vi "Super Market Billing System.vi"() -> ()   [LabVIEW 2021]
panel:
  in  "Tab Control":enum32{"Page 1", "Page 2"}(tab)
  in  "Refresh Button":bool
  in  "Password":string
  in  "User Name":string
  out "Result":dbl
  in  "Number 2":dbl
  in  "Number 1":dbl
  in  "stop":bool
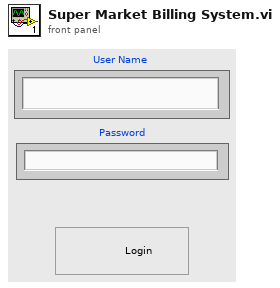
[diagram p1: front panel]
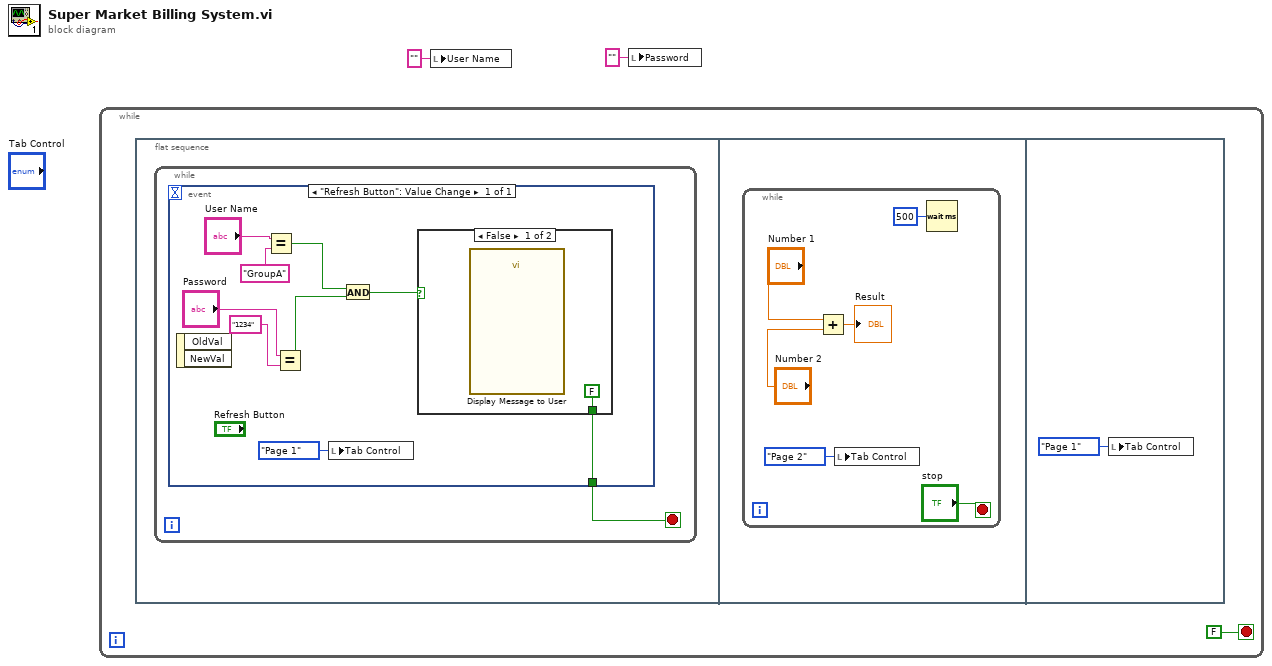
[diagram p0: block diagram]
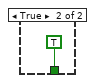
[diagram p2: hidden frame]
diagram:
  n1 = while {
    stop <- FALSE stop-if-true
    n2 = flat-sequence {
      frame #0 {
        n3 = while {
          stop <- w4 stop-if-true
          n4 = event shown="[0] \"Refresh Button\": Value Change" {
            selector: _ -> [_]
            dyn-events: _ -> [_]
            timeout: _ -> [_]
            tunnel: [w6] -> w4
            event "Refresh Button": Value Change {
              n5 = event-data() -> ()  [unwired: 1 in, 2 out]
              n6 = Equal?(x="User Name", y="GroupA") -> (x = y?=w9:bool)
              n7 = Equal?(x="Password", y="1234") -> (x = y?=w8:bool)
              n8 = local write "Tab Control"(enum32{"Page 1", "Page 2"}."Page 1" ("Tab Control")) -> ()
              n9 = And(x=w9, y=w8) -> (x .and. y?=w7:bool)
              n10 = case shown="False" w7 {
                tunnel: [FALSE TRUE] -> w6
                frame False {
                  n11 = call "Display Message to User"() -> ()  [unwired: 10 in, 2 out]
                }
                frame True {
                }
              }
            }
          }
        }
      }
      frame #1 {
        n12 = while {
          stop <- "stop" stop-if-true
          n13 = Add(x="Number 1", y="Number 2") -> (x+y=→"Result":dbl)
          n14 = local write "Tab Control"(enum32{"Page 1", "Page 2"}."Page 2" ("Tab Control")) -> ()
          n15 = Wait (ms)(milliseconds to wait=u32 500) -> ()  [unwired: 1 out]
        }
      }
      frame #2 {
        n16 = local write "Tab Control"(enum32{"Page 1", "Page 2"}."Page 1" ("Tab Control")) -> ()
      }
    }
  }
  n17 = local write "User Name"("" ("User Name")) -> ()
  n18 = local write "Password"("" ("Password")) -> ()
